vi "Digital Output.vi"(10 "DO State":bool, 11 "DIO Channel":T1=enum."DIO 1") -> ()   [LabVIEW 2016]
uses:
  <vilib>/Rock Robotics/SystemInterfaces/DIO/FPGA_DIOChannel.ctl
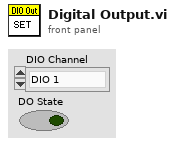
[diagram p1: front panel]
types:
  T1 = typedef "FPGA_DIOChannel.ctl" = enum8{"DIO 0", "DIO 1", "DIO 2", "DIO 3", "DIO 4", "DIO 5", "DIO 6", "DIO 7", "DIO 8", "DIO 9", "DIO MXP 0", "DIO MXP 1", "DIO MXP 2", "DIO MXP 3", "DIO MXP 4", "DIO MXP 5", "DIO MXP 6", "DIO MXP 7", "DIO MXP 8", "DIO MXP 9", "DIO MXP 10", "DIO MXP 11", "DIO MXP 12", "DIO MXP 13", "DIO MXP 14", "DIO MXP 15", "SPI Port CS1", "SPI Port CS2", "SPI Port CS3", "SPI Port MISO", "SPI Port MOSI", "Invalid"}
  T2 = typedef "WPI_DigitalOutputDevRef.ctl" = cluster{"DIO Channel":T1, "DevStatus":errorcluster}
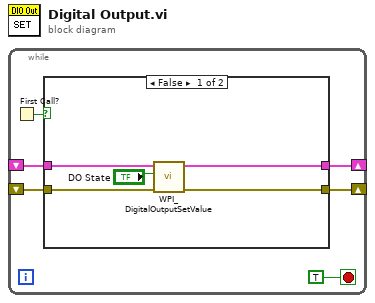
[diagram p0: block diagram]
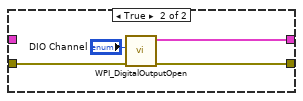
[diagram p2: hidden frame]
diagram:
  n1 = while {
    shift-right: [w4] -> _
    shift-left: _ -> [w3]
    shift-right: [w2] -> _
    shift-left: _ -> [w1]
    stop <- TRUE stop-if-true
    n2 = First Call?() -> (First Call?: T/F=w5:bool)
    n3 = case shown="False" w5 {
      tunnel: [w10 w15] -> w4
      tunnel: w3 -> [w11 w14]
      tunnel: [w9 w12] -> w2
      tunnel: w1 -> [w8 _]
      frame False {
        n4 = call <vilib>:"WPI_DigitalOutputSetValue.vi"("error in (no error)"=w11, "Value"="DO State", "DigitalOutputDevRef"=w8) -> ("error out"=w10:errorcluster, "DigitalOutputDevRef"=w9:T2)  [unwired: 7 in]
      }
      frame True {
        n5 = call <vilib>:"WPI_DigitalOutputOpen.vi"("error in (no error)"=w14, "DIO Channel"="DIO Channel") -> ("error out"=w15:errorcluster, "DigitalOutputDevRef"=w12:T2)  [unwired: 8 in]
      }
    }
  }
